vi "SubVI_Overlay Line(Fit Line & Perpendicular)#.vi"(7 "Overlay Result":bool, 8 "Perpendicular Line(Offset)":T1, 9 "Fit Line(Offset)":T1, 10 "Result":cluster{"Name":string, "NG?":bool, "Score":dbl}, 11 "Image Src In":T2) -> ()   [LabVIEW 2013]
uses:
  <vilib>/vision/Image Controls.llb/IMAQ Image.ctl
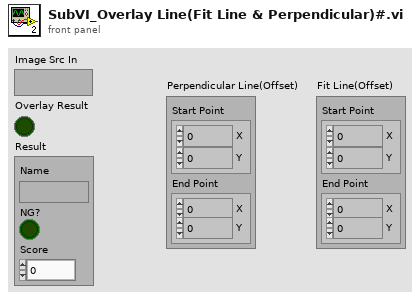
[diagram p1: front panel]
types:
  T1 = cluster{"Start Point":cluster{"X":i32, "Y":i32}, "End Point":cluster{"X":i32, "Y":i32}}
  T2 = typedef "IMAQ Image.ctl" = refnum<image>
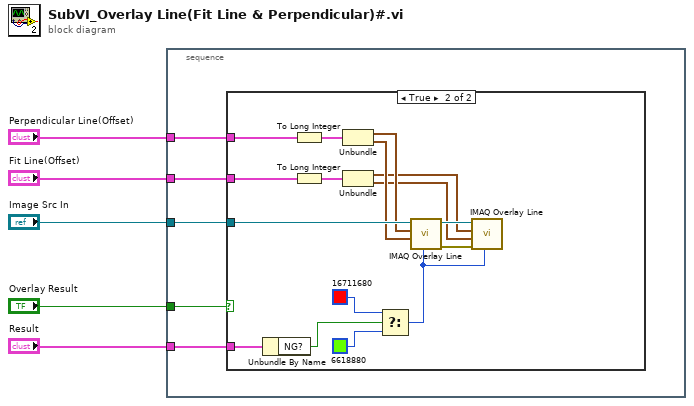
[diagram p0: block diagram]
diagram:
  n1 = stacked-sequence {
    tunnel: "Image Src In" -> [w8]
    tunnel: "Overlay Result" -> [w10]
    tunnel: "Result" -> [w9]
    tunnel: "Perpendicular Line(Offset)" -> [w7]
    tunnel: "Fit Line(Offset)" -> [w6]
    frame #0 {
      n2 = case shown="True" w10 {
        tunnel: w8 -> [_ w24]
        tunnel: w9 -> [_ w23]
        tunnel: w7 -> [_ w18]
        tunnel: w6 -> [_ w17]
        frame False {
        }
        frame True {
          n3 = Unbundle By Name(w23) -> ("NG?"=w22:bool)
          n4 = To Long Integer(number=w18) -> (32bit integer=w16:T1)
          n5 = To Long Integer(number=w17) -> (32bit integer=w15:T1)
          n6 = Unbundle(w16) -> ("Start Point"=w14:cluster{"X":i32, "Y":i32}, "End Point"=w13:cluster{"X":i32, "Y":i32})
          n7 = Unbundle(w15) -> ("Start Point"=w12:cluster{"X":i32, "Y":i32}, "End Point"=w11:cluster{"X":i32, "Y":i32})
          n8 = Select(t=u32 16711680 ("Color"), s=w22, f=u32 6618880 ("Color")) -> (s? t:f=w19:u32)
          n9 = call "IMAQ Overlay Line"("Color"=w19, "End Point"=w13, "Start Point"=w14, "Image"=w24) -> ("error out"=w26:errorcluster, "Image Out"=w25:T2)  [unwired: 6 in]
          n10 = call "IMAQ Overlay Line"("Color"=w19, "error in (no error)"=w26, "End Point"=w11, "Start Point"=w12, "Image"=w25) -> ()  [unwired: 5 in, 2 out]
        }
      }
    }
  }
